vi "Settings.vi"(4 "Baseplate Tray ID":i32, 6 "Sensor Tray ID":i32, 7 "Glue step":enum16{"Kapton", "Sensor", "PCB"}(ring), 8 "error in (no error)":errorcluster, 9 "Gantry Region":i32=1, 10 "Position Number":i32=1, 11 "Baseplate Tray In":refnum<class "Assembly Tray.lvclass">) -> (0 "error out":errorcluster, 3 "Baseplate Tray Out":refnum<class "Assembly Tray.lvclass">)   [LabVIEW 2016, in "Assembly Tray.lvclass"]
uses:
  Assembly Tray.lvclass
  C:/Users/HEP Gantry/Documents/GitHub/UCSB-Gantry/V5/Classes/Workspace/Fixture.lvclass
  Assembly Tray.lvclass/Assembly Tray.ctl
  Fixture.lvclass/Fixture.ctl
  Write Gantry Region.vi
  Write Position.vi
  Write Fixture ID.vi
panel:
  in  "Component Thickness":dbl=2.0 format="%#_13g"
  in  "Tray Number":i32=1
  # "Baseplate Tray"
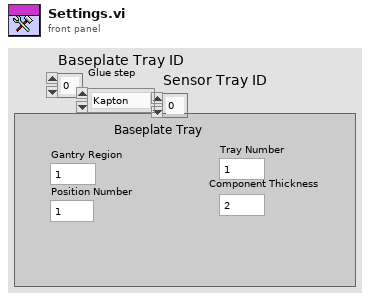
[diagram p1: front panel]
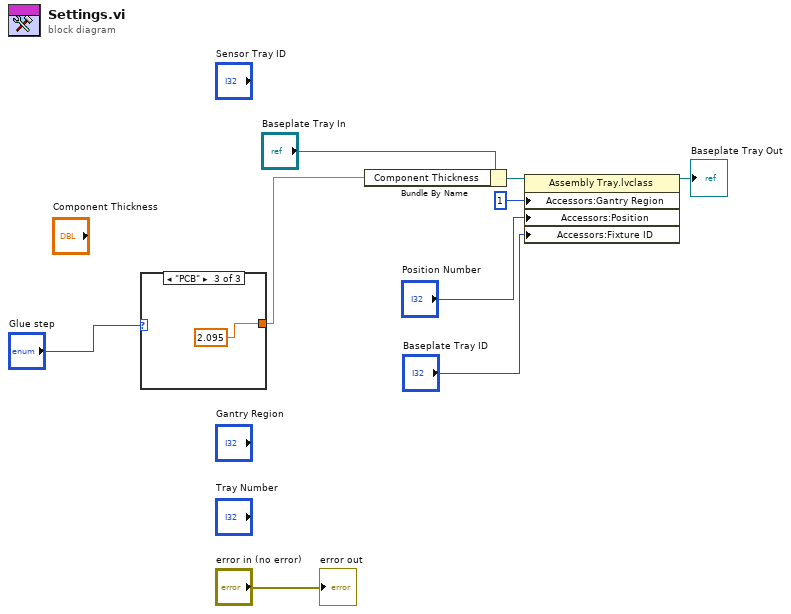
[diagram p0: block diagram]
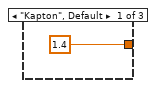
[diagram p2: hidden frame]
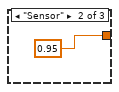
[diagram p3: hidden frame]
diagram:
  n1 = case shown="\"PCB\"" "Glue step" {
    tunnel: [1.4 0.95 2.095] -> w1
    frame "Kapton", Default {
    }
    frame "Sensor" {
    }
    frame "PCB" {
    }
  }
  n2 = Bundle By Name(cluster="Baseplate Tray In", "Component Thickness"=w1) -> (w6:refnum<class "Assembly Tray.lvclass">)
  n3 = property class="Assembly Tray.lvclass"(reference=w6, "Accessors:Gantry Region"=1, "Accessors:Position"="Position Number", "Accessors:Fixture ID"="Baseplate Tray ID") -> (reference out=→"Baseplate Tray Out":refnum<class "Assembly Tray.lvclass">)  [unwired: 1 in, 1 out]
  "error out" <- "error in (no error)"
